vi "ClassLineWithNotifier.vi"() -> ()   [LabVIEW 2012]
uses:
  DataBank/DataBank.lvclass
  DataBank/DataBank.lvclass/DataBank.ctl
panel:
  out "DataInStep4":T1
  out "DataInStep3InLine2":T1
  out "DataInStep3":T1
  out "DataInStep2":T1
  out "DataInStep1":T1
  # "請見方塊圖說明"
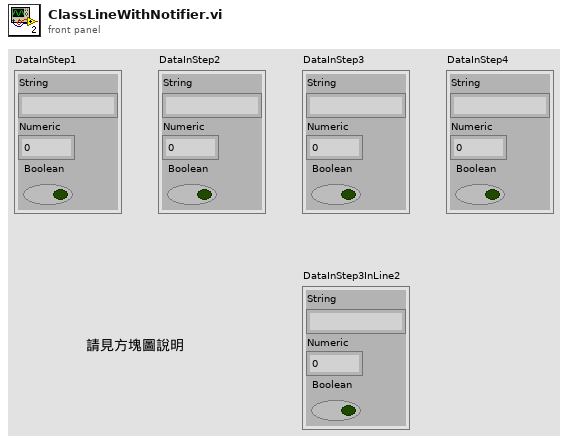
[diagram p1: front panel]
types:
  T1 = cluster{"String":string, "Numeric":i32, "Boolean":bool}
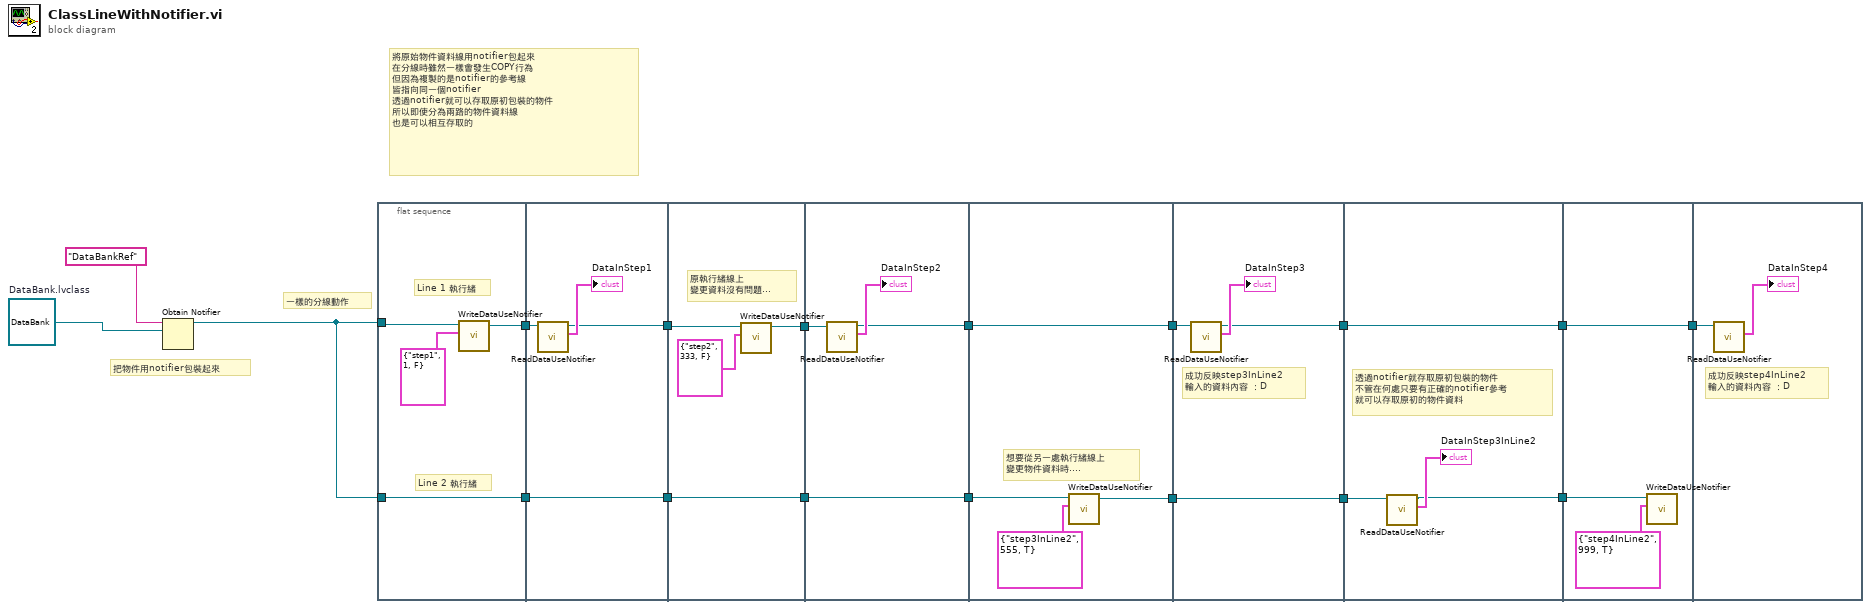
[diagram p0: block diagram]
diagram:
  w7 = refnum<class "DataBank.lvclass"> refnum  # DataBank.lvclass
  # "把物件用notifier包裝起來"
  # "將原始物件資料線用notifier包起來\n在分線時雖然一樣會發生COPY行為\n但因為複製的是notifier的參考線\n皆指向同一個notifier\n透過notifier就可以存取原初包裝的物件\n所以即使分為兩路的物件資料線\n也是可以相互存取的"
  # "一樣的分線動作"
  n1 = Obtain Notifier(name (unnamed)="DataBankRef", notification data type=w7) -> (notifier out=w5:refnum<notifier>)  [unwired: 2 in, 2 out]
  n2 = flat-sequence {
    tunnel: w5 -> [w22]
    tunnel: [w20] -> w18
    tunnel: [w19] -> w14
    tunnel: w5 -> [w19]
    tunnel: w18 -> [w26]
    tunnel: [w24] -> w17
    tunnel: [w23] -> w16
    tunnel: w14 -> [w23]
    tunnel: w17 -> [w29]
    tunnel: w16 -> [w27]
    tunnel: [w28] -> w15
    tunnel: [w27] -> w12
    tunnel: w15 -> [w33]
    tunnel: [w32] -> w13
    tunnel: w12 -> [w32]
    tunnel: [w31] -> w11
    tunnel: w13 -> [w37]
    tunnel: w11 -> [w36]
    tunnel: [w36] -> w10
    tunnel: [w35] -> w9
    tunnel: w10 -> [w41]
    tunnel: w9 -> [w40]
    tunnel: [w40] -> w8
    tunnel: [w39] -> w1
    tunnel: w8 -> [w45]
    tunnel: [w44] -> w4
    tunnel: [w43] -> w2
    tunnel: w1 -> [w43]
    tunnel: w4 -> [w48]
    tunnel: [w47] -> w3
    tunnel: w2 -> [w47]
    tunnel: w3 -> [w50]
    frame #0 {
      # "Line 2 執行緒"
      # "Line 1 執行緒"
      n3 = call "WriteDataUseNotifier.vi"("Data"=T1 {"String"="step1", "Numeric"=1, "Boolean"=FALSE}, "notifier out"=w22) -> ("notifier out"=w20:refnum<notifier>)  [unwired: 8 in, 1 out]
    }
    frame #1 {
      n4 = call "ReadDataUseNotifier.vi"("notifierIn"=w26) -> ("Data"=→"DataInStep1":T1, "notifier out"=w24:refnum<notifier>)  [unwired: 8 in, 1 out]
    }
    frame #2 {
      # "原執行緒線上\n變更資料沒有問題..."
      n5 = call "WriteDataUseNotifier.vi"("Data"=T1 {"String"="step2", "Numeric"=333, "Boolean"=FALSE}, "notifier out"=w29) -> ("notifier out"=w28:refnum<notifier>)  [unwired: 8 in, 1 out]
    }
    frame #3 {
      n6 = call "ReadDataUseNotifier.vi"("notifierIn"=w33) -> ("Data"=→"DataInStep2":T1, "notifier out"=w31:refnum<notifier>)  [unwired: 8 in, 1 out]
    }
    frame #4 {
      # "想要從另一處執行緒線上\n變更物件資料時...."
      n7 = call "WriteDataUseNotifier.vi"("Data"=T1 {"String"="step3InLine2", "Numeric"=555, "Boolean"=TRUE}, "notifier out"=w37) -> ("notifier out"=w35:refnum<notifier>)  [unwired: 8 in, 1 out]
    }
    frame #5 {
      # "成功反映step3InLine2\n輸入的資料內容 ：D"
      n8 = call "ReadDataUseNotifier.vi"("notifierIn"=w41) -> ("Data"=→"DataInStep3":T1, "notifier out"=w39:refnum<notifier>)  [unwired: 8 in, 1 out]
    }
    frame #6 {
      # "透過notifier就存取原初包裝的物件\n不管在何處只要有正確的notifier參考\n就可以存取原初的物件資料"
      n9 = call "ReadDataUseNotifier.vi"("notifierIn"=w45) -> ("Data"=→"DataInStep3InLine2":T1, "notifier out"=w44:refnum<notifier>)  [unwired: 8 in, 1 out]
    }
    frame #7 {
      n10 = call "WriteDataUseNotifier.vi"("Data"=T1 {"String"="step4InLine2", "Numeric"=999, "Boolean"=TRUE}, "notifier out"=w48) -> ()  [unwired: 8 in, 2 out]
    }
    frame #8 {
      # "成功反映step4InLine2\n輸入的資料內容 ：D"
      n11 = call "ReadDataUseNotifier.vi"("notifierIn"=w50) -> ("Data"=→"DataInStep4":T1)  [unwired: 8 in, 2 out]
    }
  }
